vi "get index definition.vi"(10 "channel classification":T1, 11 "Temperature Chamber Model configuration in":refnum<class "Temperature Chamber Model configuration.lvclass">) -> (1 "valid?":bool, 2 "index cluster":variant, 3 "Temperature Chamber Model configuration out":refnum<class "Temperature Chamber Model configuration.lvclass">)   [LabVIEW 2015, in "Temperature Chamber Model configuration.lvclass"]
uses:
  Temperature Chamber Model configuration.lvclass
  <vilib>/NI/Tag Bus Module Framework/channel/channel classification.ctl
  parameter data indices.ctl
  result data indices.ctl
  <vilib>/NI/Tag Bus Module Framework/channel/TBM channel.lvclass
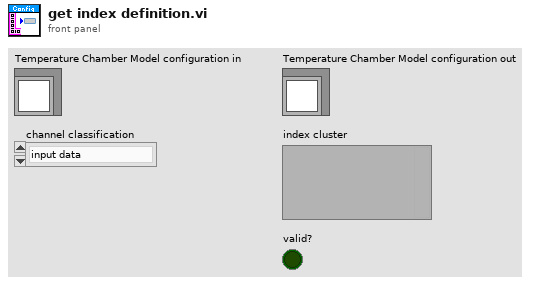
[diagram p1: front panel]
types:
  T1 = typedef "TBM channel.lvclass/channel classification.ctl" = enum16{"input data", "output data", "processing parameter", "processing result"}
  T2 = typedef "Temperature Chamber Model configuration.lvclass/parameter data indices.ctl" = cluster{"Double.Ambient Temperature":i32, "Double.Fan PWM":i32, "Double.Lamp PWM":i32}
  T3 = typedef "Temperature Chamber Model configuration.lvclass/result data indices.ctl" = cluster{"Double.Thermocouple Reading":i32}
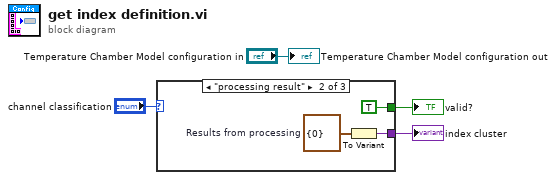
[diagram p0: block diagram]
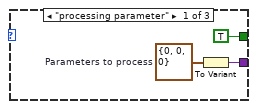
[diagram p2: hidden frame]
diagram:
  n1 = case shown="\"processing result\"" "channel classification" {
    tunnel: [TRUE TRUE _] -> w2
    tunnel: [w6 w9 _] -> w1
    frame "processing parameter" {
      w5 = T2 {"Double.Ambient Temperature"=0, "Double.Fan PWM"=0, "Double.Lamp PWM"=0}  # Parameters to process
      n2 = To Variant(anything=w5) -> (Variant=w6:variant)
    }
    frame "processing result" {
      w8 = T3 {"Double.Thermocouple Reading"=0}  # Results from processing
      n3 = To Variant(anything=w8) -> (Variant=w9:variant)
    }
    frame Default {
    }
  }
  "valid?" <- w2
  "index cluster" <- w1
  "Temperature Chamber Model configuration out" <- "Temperature Chamber Model configuration in"
